vi "InstrumentControlExercises_MichaelVasmerDavidWise.vi"() -> ()   [LabVIEW 2012]
doc: "This example shows how to configure a measurement and take a reading."
uses:
  Program Files/National Instruments/LabVIEW 2014/instr.lib/Keithley 24XX/Keithley 24XX.lvlib
  <vilib>/express/express arith-compare/Formula/XNode/ExpressFormulaBlockNode.xnode
  Control2_MichaelVasmerDavidWise.ctl
  He3_Tlogger_Global 1.vi
  Control3_MichaelVasmerDavidWise.ctl
  Program Files/National Instruments/LabVIEW 2014/instr.lib/Stanford Research 830/Stanford Research 830.lvlib
  Program Files/National Instruments/LabVIEW 2014/instr.lib/Keithley 24XX/Public/Data/Read (Single Point).vi
  Program Files/National Instruments/LabVIEW 2014/instr.lib/Stanford Research 830/Public/Data/Read (All Parameters).vi
  <vilib>/Utility/file.llb/Write To Spreadsheet File (string).vi
  <vilib>/Utility/file.llb/Write To Spreadsheet File (DBL).vi
panel:
  out "T 2":dbl
  out "T 1":dbl
  out "Resistance(T) vs Time":dbl(graph)
  out "Resistance(B) vs Time":dbl(graph)
  out "V_output_Y_channel":dbl
  out "V_output_X_channel":dbl
  in  "R Series Value":dbl=100000.0
  in  "File String Template 2":string
  in  "File String Template":string
  in  "True  = R(B)\nFalse = R(T)":bool
  in  "Lock In On (default false)":bool
  out "Outer State Machine":T1=enum."Idle"
  in  "Force Measurement":bool
  out "Inner State Machine":T2=enum."Open File"
  out "I_AC Amplitude (A)":dbl=1.0
  in  "Keithley on (default false)":bool
  out "Magnetic Field (T)":dbl
  in  "Internal Reference Frequency (1000 Hz)":dbl=1000.0
  in  "Sine Output Amplitude (1 V)":dbl=1.0
  in  "Sensitivity (26: 1 V/uA)":i8(ring)=26 items=["Auto Gain"=-1, "2 nV/fA"=0, "5 nV/fA"=1, "10 nV/fA"=2, "20 nV/fA"=3, "50 nV/fA"=4, "100 nV/fA"=5, "200 nV/fA"=6, "500 nV/fA"=7, "1 uV/pA"=8, "2 uV/pA"=9, "5 uV/pA"=10, "10 uV/pA"=11, "20 uV/pA"=12, "50 uV/pA"=13, "100 uV/pA"=14, "200 uV/pA"=15, "500 uV/pA"=16, "1 mV/nA"=17, "2 mV/nA"=18, "5 mV/nA"=19, "10 mV/nA"=20, "20 mV/nA"=21, "50 mV/nA"=22, "100 mV/nA"=23, "200 mV/nA"=24, "500 mV/mA"=25, "1 V/uA"=26]
  in  "Dynamic Reserve (2: Low Noise)":i8(ring)=2 items=["High Reserve"=0, "Normal"=1, "Low Noise"=2, "Auto Reserve"=-1]
  in  "Reference Source (1: Internal)":u16(ring)=1 items=["External", "Internal"]
  in  "Input Coupling (0: AC)":u16(ring) items=["AC", "DC"]
  in  "Input Connection (0: Single-Ended Voltage)":u16(ring) items=["Single-Ended Voltage", "Differential Voltage", "1 MOhm Current Gain", "100 MOhm Current Gain"]
  in  "VISA resource name Lock-In":refnum<visa-resource-name>
  in  "Stop Sweep R(T)":bool
  in  "Sweep R(T)":bool
  out "Temperature (K)":dbl
  in  "Shutdown":bool
  in  "B Max\n|B|<0.0716":dbl
  in  "Sweep R(B)":bool
  in  "Steps":dbl
  out "Field too high error":string
  in  "Compliance  Level (0.1)":dbl=0.1
  out "Resistance":sgl
  out "Current":sgl
  out "Voltage":sgl
  in  "Enable Resistance Auto Range (T:Enable)":bool=TRUE
  in  "Enable Current Auto Range (T:Enable)":bool=TRUE
  in  "Enable Voltage Auto Range (T:Enable)":bool=TRUE
  in  "Resistance Manual Range (1.0)":dbl=1.0
  in  "Current Manual Range (1.0)":dbl=1.0
  in  "Voltage Manual Range (1.0)":dbl=1.0
  in  "Serial Configuration":T3={"Baud Rate"=9600, "Parity"=0, "Data Bits"=8, "Stop Bits"=10, "Flow Control"=0} {"Flow Control" items=["None", "XON/XOFF", "RTS/CTS", "XON/XOFF & RTS/CTS", "DTR/DSR", "XON/XOFF & DTR/DSR"]; "Stop Bits" items=["1.0"=10, "1.5"=15, "2.0"=20]; "Data Bits" items=["7"=7, "8"=8]; "Parity" items=["None", "Odd", "Even", "Mark", "Space"]; "Baud Rate" items=["300"=300, "600"=600, "1200"=1200, "2400"=2400, "4800"=4800, "9600"=9600, "19200"=19200]}
  in  "VISA resource name Kiethley":refnum<visa-resource-name>
  # "Keithley Settings"
  # "Voltage Range Settings"
  # "Current Range Settings"
  # "Resistance Range Settings"
  # "Keithley Output"
  # "SR830 Lock In Settings"
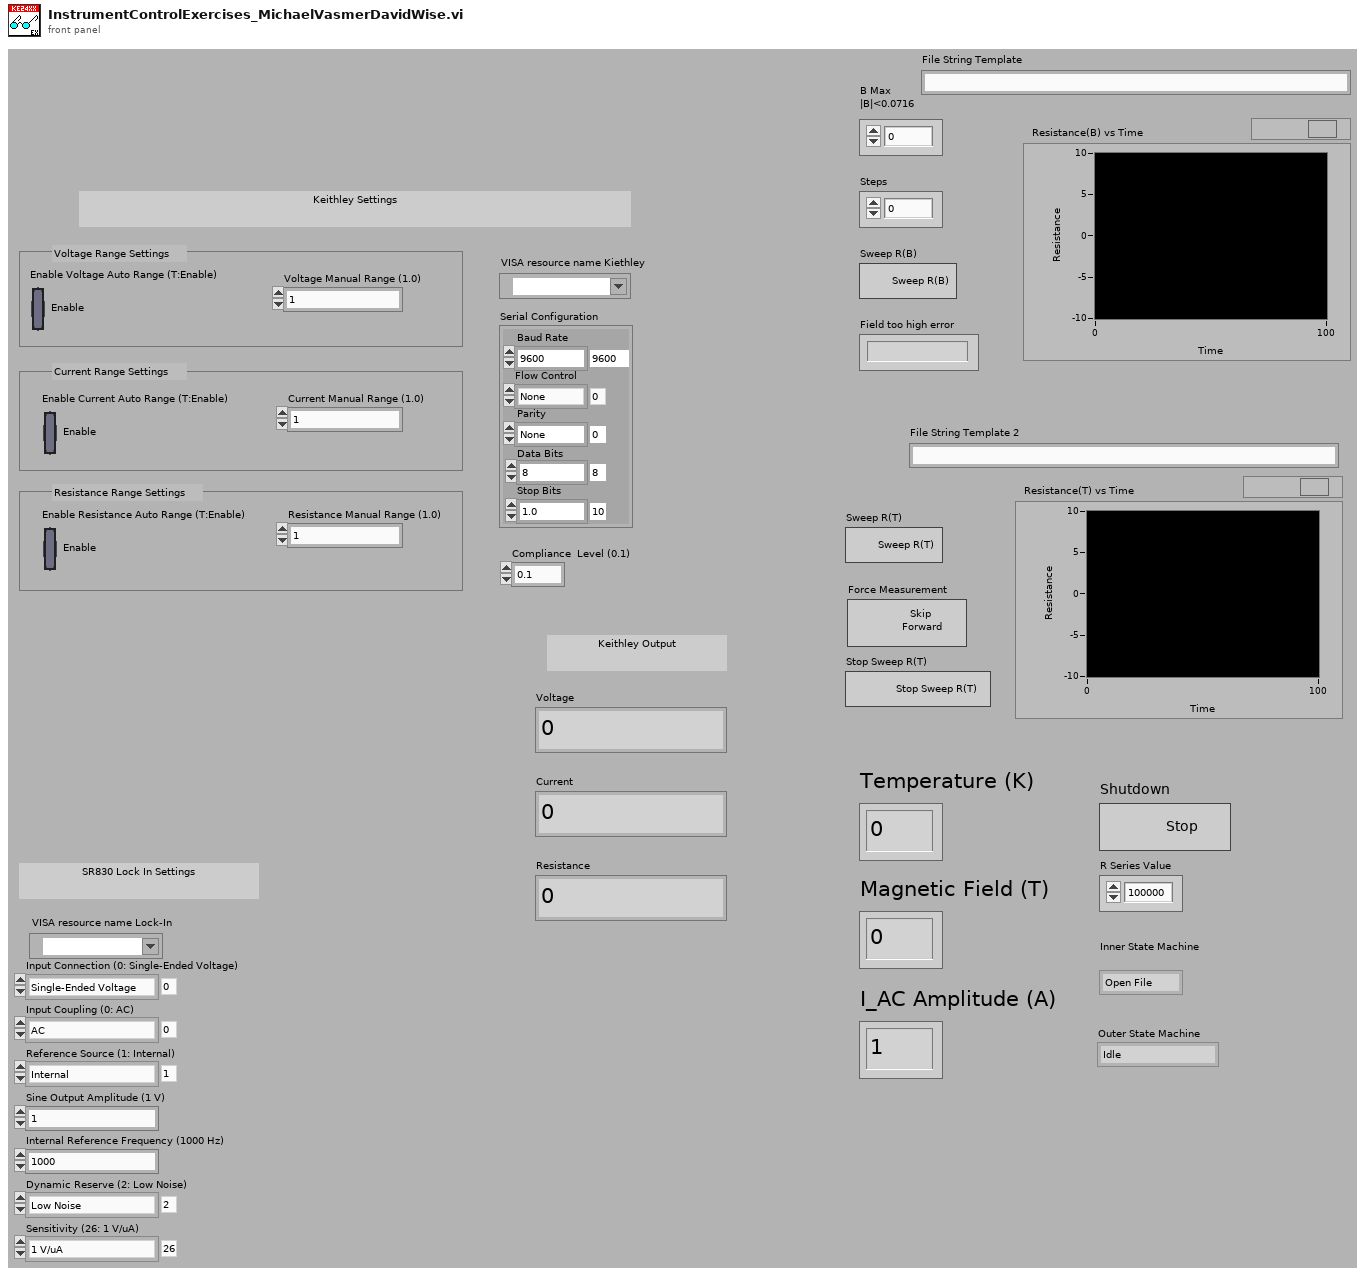
[diagram p1: front panel]
types:
  T1 = typedef "Control2_MichaelVasmerDavidWise.ctl" = enum16{"Write File", "Open File", "Shutdown All", "Shutdown Lock in", "Read R(T)", "Init Lock In", "Increment", "Shutdown Keithley", "Idle", "Exit", "Read R(B)", "Set B", "Init Keithley"}
  T2 = typedef "Control3_MichaelVasmerDavidWise.ctl" = enum16{"Write File", "Open File", "Read T 2", "Idle", "Read Lockin", "Read T"}
  T3 = cluster{"Baud Rate":u32, "Parity":u16, "Data Bits":u16, "Stop Bits":u16, "Flow Control":u16}
  T4 = cluster{"X-Value":dbl, "Y-Value":dbl, "R-Value":dbl, "Theta-Value":dbl, "Aux In 1 Value":dbl, "Aux In 2 Value":dbl, "Aux In 3 Value":dbl, "Aux In 4 Value":dbl, "Reference Frequency":dbl, "Channel 1 Display":dbl, "Channel 2 Display":dbl}
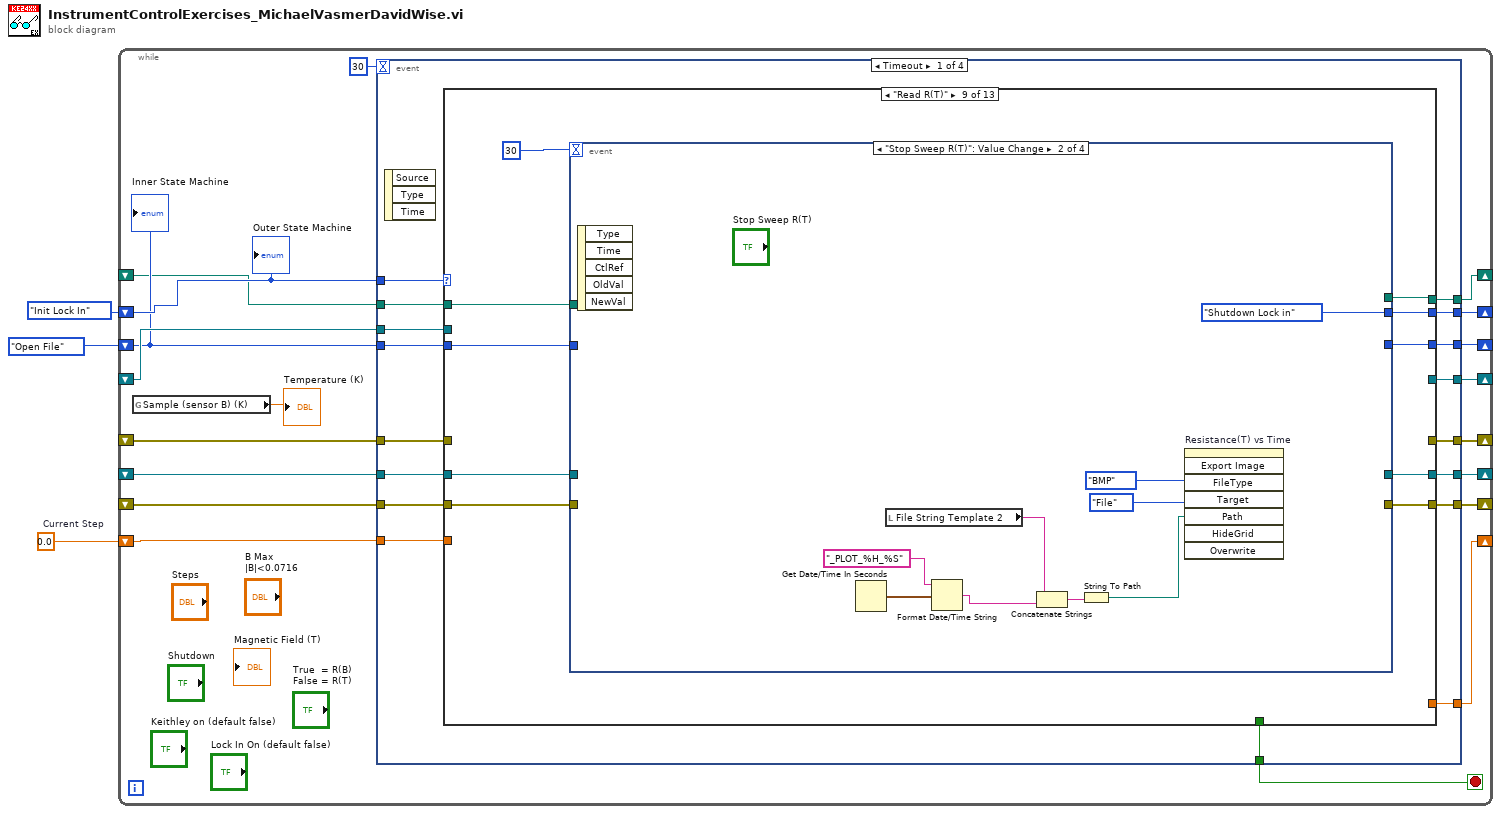
[diagram p0: block diagram]
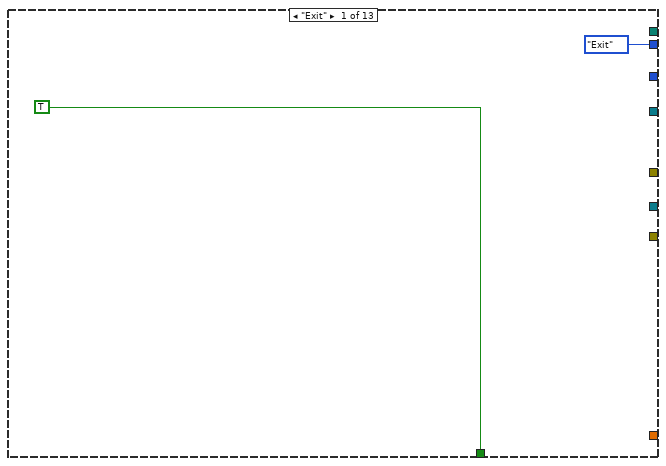
[diagram p2: hidden frame]
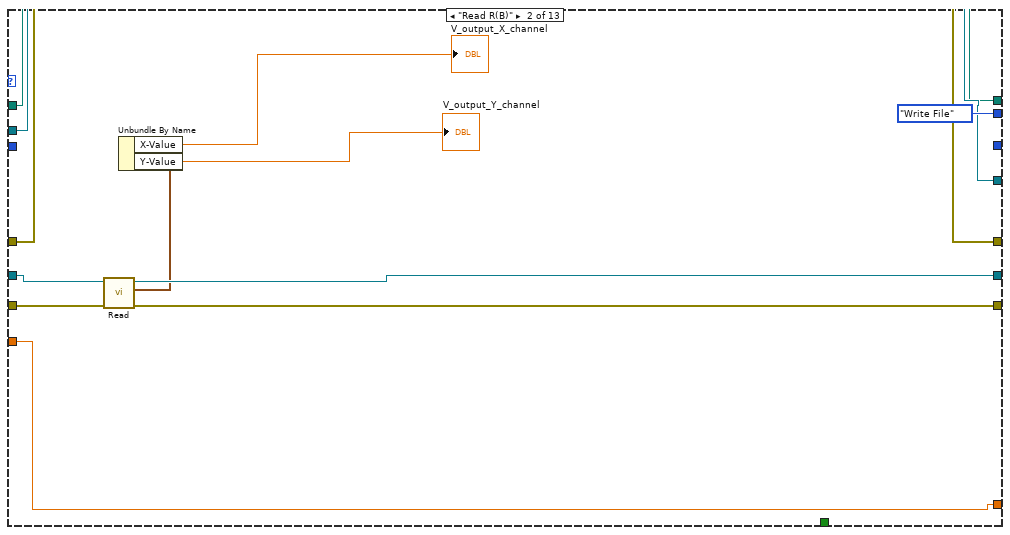
[diagram p3: hidden frame]
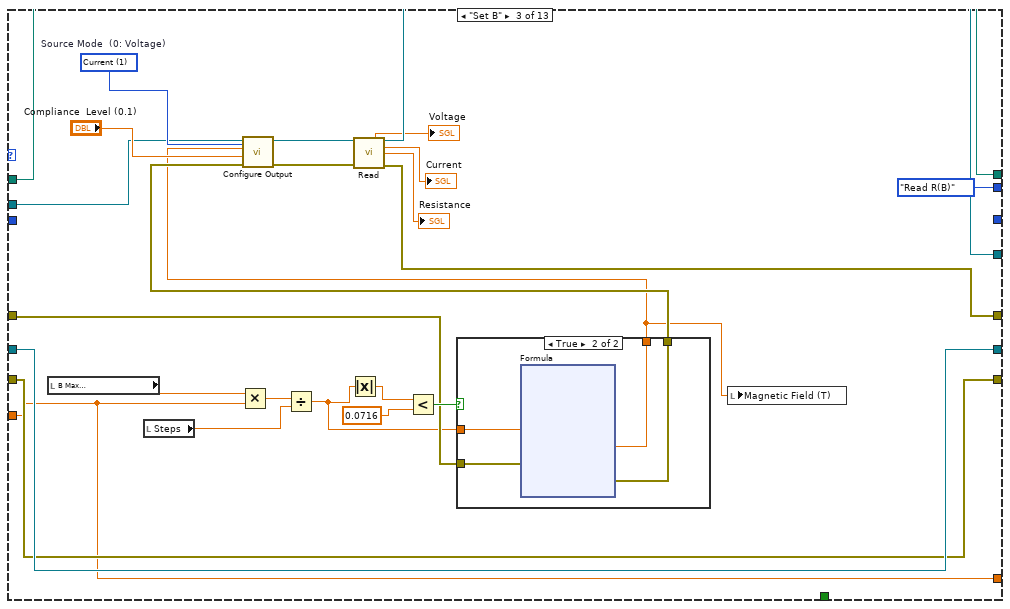
[diagram p4: hidden frame]
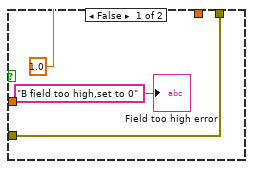
[diagram p5: hidden frame]
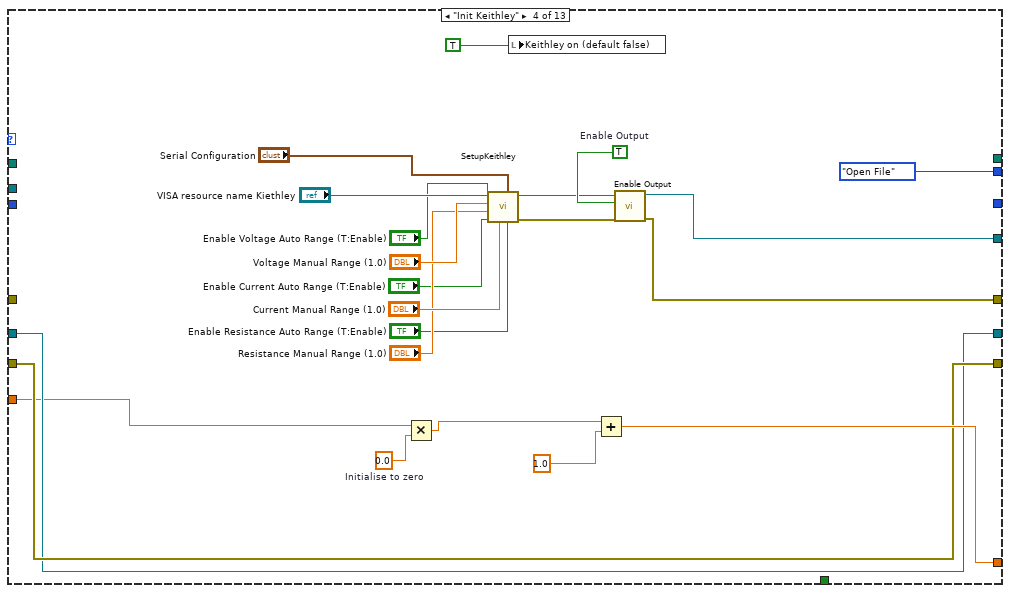
[diagram p6: hidden frame]
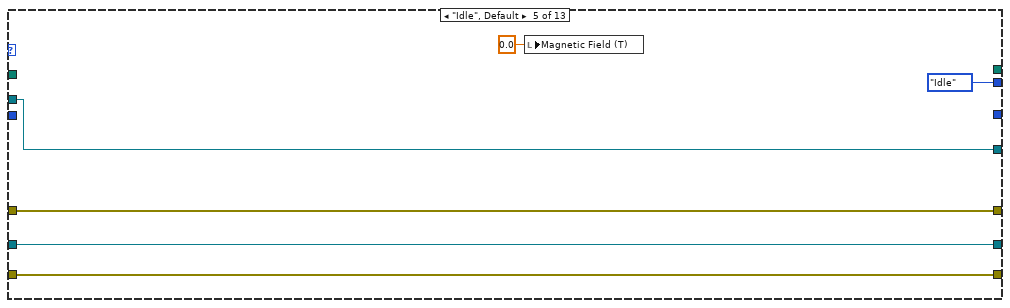
[diagram p7: hidden frame]
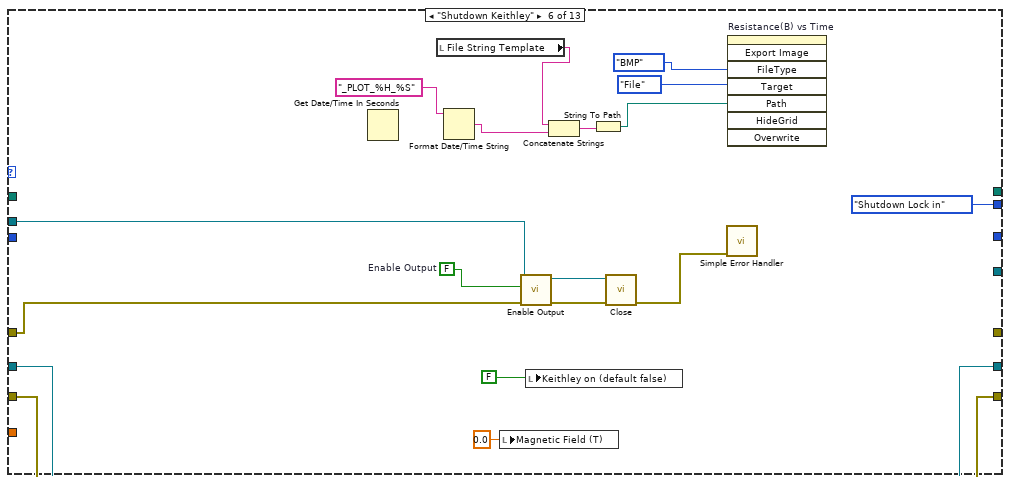
[diagram p8: hidden frame]
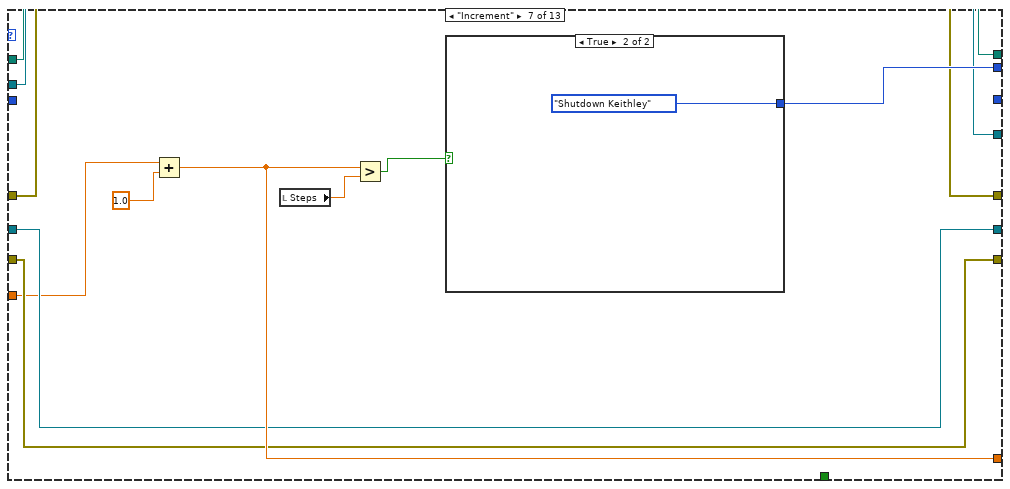
[diagram p9: hidden frame]
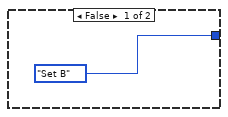
[diagram p10: hidden frame]
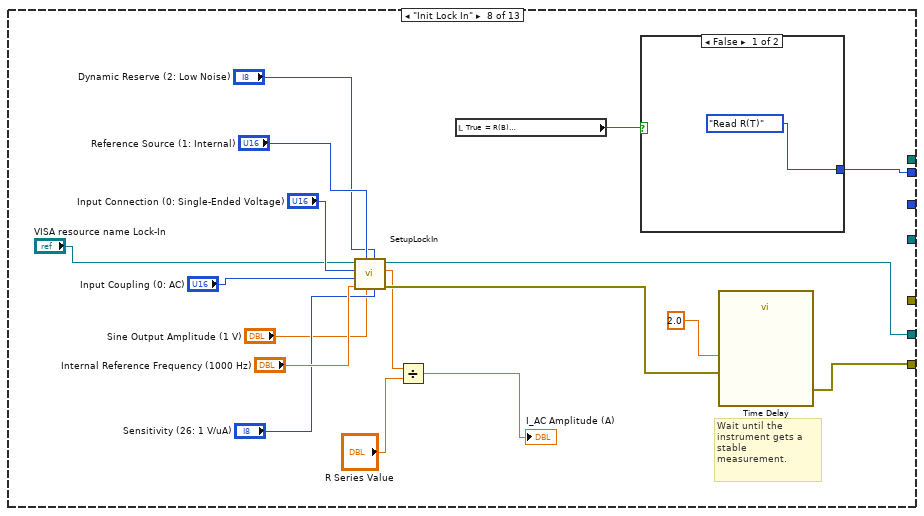
[diagram p11: hidden frame]
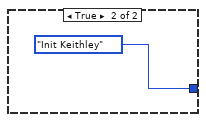
[diagram p12: hidden frame]
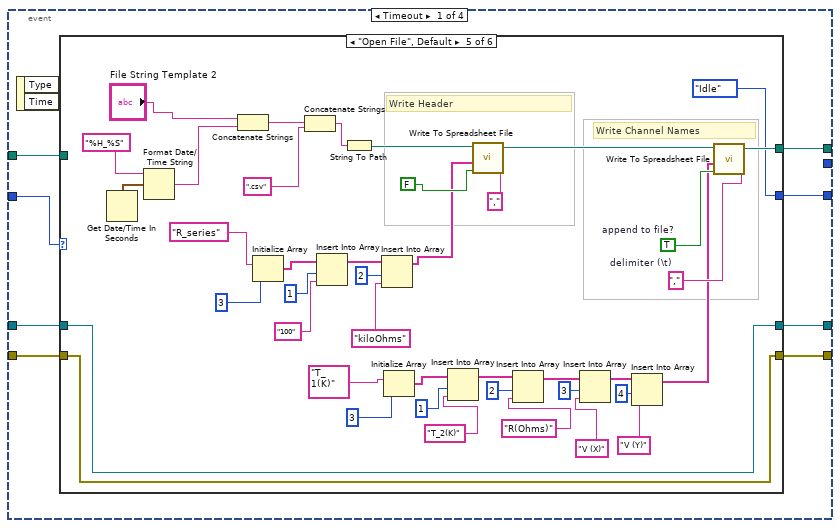
[diagram p13: hidden frame]
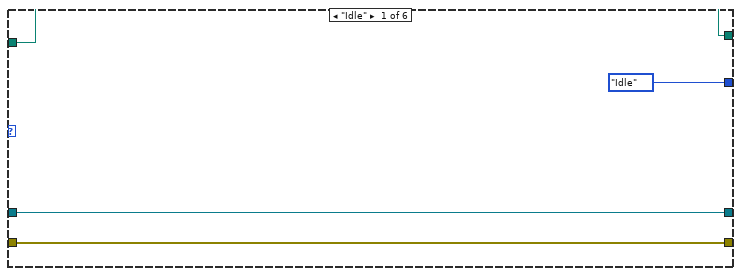
[diagram p14: hidden frame]
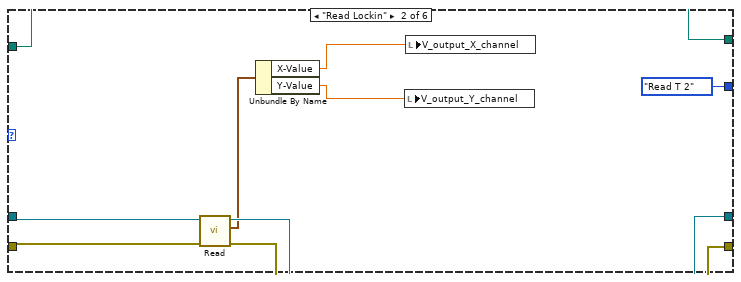
[diagram p15: hidden frame]
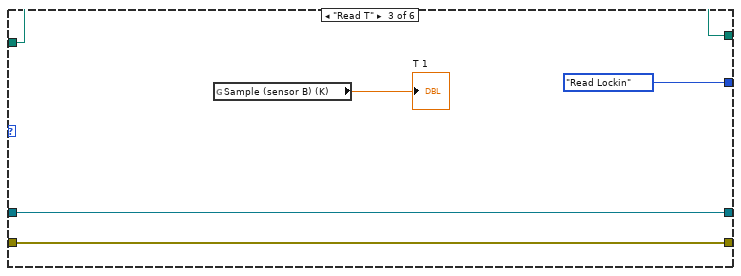
[diagram p16: hidden frame]
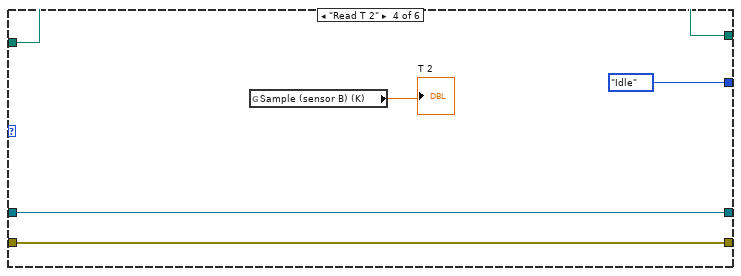
[diagram p17: hidden frame]
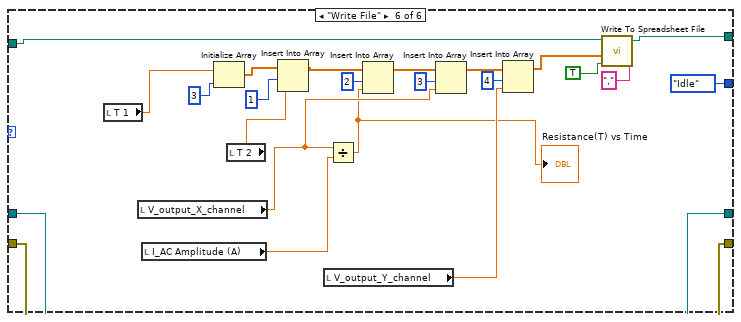
[diagram p18: hidden frame]
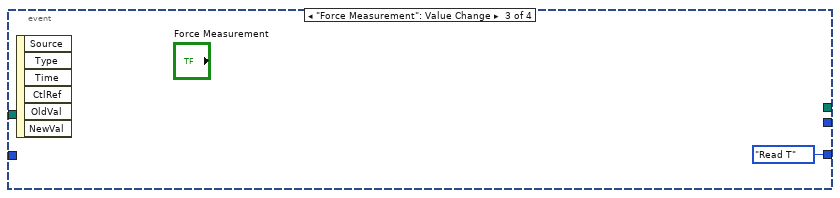
[diagram p19: hidden frame]
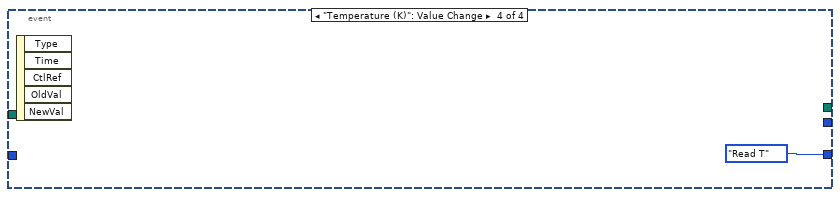
[diagram p20: hidden frame]
diagram:
  w2 = 0.0  # Current Step
  n1 = while {
    shift-right: [w21] -> _
    shift-left: Control2_MichaelVasmerDavidWise."Init Lock In" -> [w22]
    shift-right: [w20] -> _
    shift-left: _ -> [w17]
    shift-right: [w19] -> _
    shift-left: _ -> [w16]
    shift-right: [w14] -> _
    shift-left: w2 -> [w4]
    shift-right: [w13] -> _
    shift-left: Control3_MichaelVasmerDavidWise."Open File" -> [w7]
    shift-right: [w12] -> _
    shift-left: _ -> [w9]
    shift-right: [w11] -> _
    shift-left: _ -> [w10]
    shift-right: [w6] -> _
    shift-left: _ -> [w5]
    stop <- w15 stop-if-true
    n2 = global read "He3_Tlogger_Global 1.vi" "Sample (sensor B) (K)"() -> (→"Temperature (K)":dbl)
    n3 = event shown="[0] Timeout" {
      selector: _ -> [_ _ _ _]
      dyn-events: _ -> [_ _ _ _]
      timeout: 30 -> [_ _ _ _]
      tunnel: w22 -> [w39 _ _ _]
      tunnel: [w38 Control2_MichaelVasmerDavidWise."Shutdown All" Control2_MichaelVasmerDavidWise."Init Lock In" Control2_MichaelVasmerDavidWise."Init Lock In"] -> w21
      tunnel: [w37 _ _ _] -> w20
      tunnel: [w36 _ _ _] -> w19
      tunnel: w17 -> [w35 _ _ _]
      tunnel: w16 -> [w34 _ _ _]
      tunnel: [w33 _ _ _] -> w15
      tunnel: [w32 _ _ _] -> w14
      tunnel: w7 -> [w31 _ _ _]
      tunnel: [w30 _ _ _] -> w13
      tunnel: [w29 _ _ _] -> w12
      tunnel: [w28 _ _ _] -> w11
      tunnel: w10 -> [w27 _ _ _]
      tunnel: w9 -> [w26 _ _ _]
      tunnel: [w25 _ _ _] -> w6
      tunnel: w5 -> [w24 _ _ _]
      tunnel: w4 -> [w23 _ _ _]
      event Timeout {
        n4 = event-data() -> ()  [unwired: 1 in, 3 out]
        n5 = case shown="\"Read R(T)\"" w39 {
          tunnel: [Control2_MichaelVasmerDavidWise."Exit" Control2_MichaelVasmerDavidWise."Write File" Control2_MichaelVasmerDavidWise."Read R(B)" Control2_MichaelVasmerDavidWise."Open File" Control2_MichaelVasmerDavidWise."Idle" Control2_MichaelVasmerDavidWise."Shutdown Lock in" w148 w162 w178 Control2_MichaelVasmerDavidWise."Exit" _ Control2_MichaelVasmerDavidWise."Set B" Control2_MichaelVasmerDavidWise."Increment"] -> w38
          tunnel: [_ w48 w59 w107 w120 _ w146 _ _ _ _ _ w370] -> w37
          tunnel: [_ w47 w60 w99 w121 _ w145 _ _ _ _ _ w371] -> w36
          tunnel: w35 -> [_ w48 w63 _ w120 w134 w146 _ _ w291 _ _ w370]
          tunnel: w34 -> [_ w47 w61 _ w121 w138 w145 _ _ w292 _ _ w371]
          tunnel: [TRUE _ _ _ _ _ _ _ _ _ _ _ _] -> w33
          tunnel: [_ w42 w54 w103 _ _ w147 _ _ _ _ w310 w351] -> w32
          tunnel: w31 -> [_ _ _ _ _ _ _ _ w180 _ _ _ _]
          tunnel: [_ _ _ _ _ _ _ _ w179 _ _ _ _] -> w30
          tunnel: [_ w52 w67 w96 w117 w129 w143 w161 w174 _ _ _ w372] -> w29
          tunnel: [_ w51 w66 w97 w116 w130 w144 w159 w175 _ _ _ w373] -> w28
          tunnel: w27 -> [_ w50 w66 w97 w116 w130 w144 _ w177 w289 w307 _ w373]
          tunnel: w26 -> [_ w46 w67 w96 w117 w129 w143 _ w176 w290 w308 _ w372]
          tunnel: [_ w45 w55 _ _ _ w141 _ w173 _ _ w322 _] -> w25
          tunnel: w24 -> [_ w45 w55 _ _ _ w141 _ w172 _ _ _ w367]
          tunnel: w23 -> [_ w42 w54 w94 _ _ w140 _ _ _ _ w310 w351]
          frame "Exit" {
          }
          frame "Read R(B)" {
            n6 = call-poly "Read.vi"("error in (no error)"=w50, "VISA resource name"=w46) -> ("error out"=w51:errorcluster, "Parameter Values"=w49:T4, "VISA resource name out"=w52:refnum<visa-resource-name>)  [unwired: 7 in]
            n7 = Unbundle By Name(w49) -> ("X-Value"=→"V_output_X_channel":dbl, "Y-Value"=→"V_output_Y_channel":dbl)
          }
          frame "Set B" {
            w73 = u16 1 items=["Voltage", "Current"]  # Source Mode  (0: Voltage)
            n8 = local read "B Max\n|B|<0.0716"() -> (w70:dbl)
            n9 = local read "Steps"() -> (w68:dbl)
            n10 = Multiply(x=w70, y=w54) -> (x*y=w69:dbl)
            n11 = Divide(x=w69, y=w68) -> (x/y=w56:dbl)
            n12 = Absolute Value(x=w56) -> (abs(x)=w57:dbl)
            n13 = Less?(x=w57, y=0.0716 ("x")) -> (x < y?=w72:bool)
            n14 = case shown="True" w72 {
              tunnel: w56 -> [_ w85]
              tunnel: [1.0 ("x") w84] -> w62
              tunnel: w61 -> [w80 w83]
              tunnel: [w80 w82] -> w65
              frame False {
                "Field too high error" <- "B field too high,set to 0" ("String")
              }
              frame True {
                n15 = xnode "Formula"("X1"=w85, "error in (no error)"=w83) -> ("Result"=w84:dbl, "error out"=w82:errorcluster)
              }
            }
            n16 = call "Configure Output.vi"("Source Mode  (0: Voltage)"=w73, "error in (no error)"=w65, "Compliance  Level (0.1)"="Compliance  Level (0.1)", "Output Level (0)"=w62, "VISA resource name"=w63) -> ("error out"=w74:errorcluster, "VISA resource name out"=w75:refnum<visa-resource-name>)  [unwired: 5 in]
            n17 = call-poly "Read.vi"("VISA resource name"=w75, "error in (no error)"=w74) -> ("Voltage"=→"Voltage":sgl, "VISA resource name out"=w59:refnum<visa-resource-name>, "Current"=→"Current":sgl, "Resistance"=→"Resistance":sgl, "error out"=w60:errorcluster)  [unwired: 7 in, 2 out]
            n18 = local write "Magnetic Field (T)"(w62) -> ()
          }
          frame "Init Keithley" {
            w105 = 0.0  # Initialise to zero
            w108 = TRUE  # Enable Output
            n19 = Multiply(x=w94, y=w105) -> (x*y=w106:dbl)
            n20 = call "SetupKeithley.vi"("Enable Resistance Auto Range (T:Enable)"="Enable Resistance Auto Range (T:Enable)", "Serial Configuration"="Serial Configuration", "Current Manual Range (1.0)"="Current Manual Range (1.0)", "Enable Voltage Auto Range (T:Enable)"="Enable Voltage Auto Range (T:Enable)", "Enable Current Auto Range (T:Enable)"="Enable Current Auto Range (T:Enable)", "Resistance Manual Range (1.0)"="Resistance Manual Range (1.0)", "Voltage Manual Range (1.0)"="Voltage Manual Range (1.0)", "VISA Refnum in"="VISA resource name Kiethley") -> ("error out"=w100:errorcluster, "VISA Refnum out"=w98:refnum<visa-resource-name>)  [unwired: 2 in]
            n21 = local write "Keithley on (default false)"(TRUE ("Keithley on")) -> ()
            n22 = Add(x=w106, y=1.0 ("x+y")) -> (x+y=w103:dbl)
            n23 = call "Enable Output.vi"("error in (no error)"=w100, "Enable Output (T: Enable)"=w108, "VISA resource name"=w98) -> ("error out"=w99:errorcluster, "VISA resource name out"=w107:refnum<visa-resource-name>)  [unwired: 7 in]
          }
          frame "Idle", Default {
            n24 = local write "Magnetic Field (T)"(0.0 ("Magnetic Field (T)")) -> ()
          }
          frame "Shutdown Keithley" {
            w131 = FALSE  # Enable Output
            n25 = Get Date/Time In Seconds() -> ()  [unwired: 1 out]
            n26 = local read "File String Template"() -> (w123:string)
            n27 = Format Date/Time String(time format string (%c)="_PLOT_%H_%S") -> (date/time string=w122:string)  [unwired: 2 in]
            n28 = local write "Magnetic Field (T)"(0.0 ("Magnetic Field (T)")) -> ()
            n29 = call "Enable Output.vi"("error in (no error)"=w138, "Enable Output (T: Enable)"=w131, "VISA resource name"=w134) -> ("error out"=w139:errorcluster, "VISA resource name out"=w133:refnum<visa-resource-name>)  [unwired: 7 in]
            n30 = local write "Keithley on (default false)"(FALSE ("Keithley on")) -> ()
            n31 = Concatenate Strings(w123, w122) -> (w126:string)
            n32 = String To Path(string=w126) -> (path=w125:path)
            n33 = call "Close.vi"("error in (no error)"=w139, "VISA resource name"=w133) -> ("error out"=w132:errorcluster)  [unwired: 9 in]
            n34 = call <vilib>:"Simple Error Handler.vi"("error in (no error)"=w132) -> ()  [unwired: 4 in, 5 out]
            n35 = invoke on="Resistance(B) vs Time" class="WFChart (strict)" method="Export Image"("FileType"=enum32{"BMP", "EPS", "EMF", "PICT"}."BMP" ("File Type"), "Target"=enum32{"File", "Clipboard"}."File", "Path"=w125) -> ()  [unwired: 5 in, 8 out]
          }
          frame "Increment" {
            n36 = Add(x=w140, y=1.0 ("x")) -> (x+y=w147:dbl)
            n37 = local read "Steps"() -> (w149:dbl)
            n38 = Greater?(x=w147, y=w149) -> (0:w142:bool)
            n39 = case shown="True" w142 {
              tunnel: [Control2_MichaelVasmerDavidWise."Set B" Control2_MichaelVasmerDavidWise."Shutdown Keithley"] -> w148
              frame False {
              }
              frame True {
              }
            }
          }
          frame "Init Lock In" {
            # "Wait until the instrument gets a stable measurement."
            n40 = call "SetupLockIn.vi"("Sensitivity (26: 1 V/uA)"="Sensitivity (26: 1 V/uA)", "Dynamic Reserve (2: Low Noise)"="Dynamic Reserve (2: Low Noise)", "Sine Output Amplitude (1 V)"="Sine Output Amplitude (1 V)", "Reference Source (1: Internal)"="Reference Source (1: Internal)", "Internal Reference Frequency (1000 Hz)"="Internal Reference Frequency (1000 Hz)", "Input Coupling (0: AC)"="Input Coupling (0: AC)", "Input Connection (0: Single-Ended Voltage)"="Input Connection (0: Single-Ended Voltage)", "VISA Refnum in"="VISA resource name Lock-In") -> ("error out"=w160:errorcluster, "V_AC Amplitude (A)"=w155:dbl, "VISA Refnum out"=w161:refnum<visa-resource-name>)  [unwired: 1 in]
            n41 = Divide(x=w155, y="R Series Value") -> (x/y=→"I_AC Amplitude (A)":dbl)
            n42 = local read "True  = R(B)\nFalse = R(T)"() -> (w156:bool)
            n43 = case shown="False" w156 {
              tunnel: [Control2_MichaelVasmerDavidWise."Read R(T)" Control2_MichaelVasmerDavidWise."Init Keithley"] -> w162
              frame False {
              }
              frame True {
              }
            }
            n44 = call "Time Delay"("error in (no error)"=w160, "Delay Time (s)"=2.0) -> ("error out"=w159:errorcluster)  [unwired: 9 in]
          }
          frame "Read R(T)" {
            n45 = event shown="[1] \"Stop Sweep R(T)\": Value Change" {
              selector: _ -> [_ _ _ _]
              dyn-events: _ -> [_ _ _ _]
              timeout: 30 -> [_ _ _ _]
              tunnel: w180 -> [w189 _ _ _]
              tunnel: [w188 _ Control3_MichaelVasmerDavidWise."Read T" Control3_MichaelVasmerDavidWise."Read T"] -> w179
              tunnel: [_ Control2_MichaelVasmerDavidWise."Shutdown Lock in" _ _] -> w178
              tunnel: w177 -> [w187 _ _ _]
              tunnel: w176 -> [w186 _ _ _]
              tunnel: [w185 _ _ _] -> w175
              tunnel: [w184 _ _ _] -> w174
              tunnel: [w183 _ _ _] -> w173
              tunnel: w172 -> [w182 _ _ _]
              event Timeout {
                n46 = event-data() -> ()  [unwired: 1 in, 2 out]
                n47 = case shown="\"Open File\", Default" w189 {
                  tunnel: [Control3_MichaelVasmerDavidWise."Idle" Control3_MichaelVasmerDavidWise."Read T 2" Control3_MichaelVasmerDavidWise."Read Lockin" Control3_MichaelVasmerDavidWise."Idle" Control3_MichaelVasmerDavidWise."Idle" Control3_MichaelVasmerDavidWise."Idle"] -> w188
                  tunnel: w187 -> [w191 w200 w205 w210 w217 w276]
                  tunnel: w186 -> [w192 w201 w206 w211 w216 w275]
                  tunnel: [w191 w199 w205 w210 w217 w276] -> w185
                  tunnel: [w192 w198 w206 w211 w216 w275] -> w184
                  tunnel: [w190 w194 w203 w208 w220 w272] -> w183
                  tunnel: w182 -> [w190 w194 w203 w208 _ w271]
                  frame "Idle" {
                  }
                  frame "Read Lockin" {
                    n48 = call-poly "Read.vi"("error in (no error)"=w200, "VISA resource name"=w201) -> ("error out"=w199:errorcluster, "Parameter Values"=w197:T4, "VISA resource name out"=w198:refnum<visa-resource-name>)  [unwired: 7 in]
                    n49 = Unbundle By Name(w197) -> ("X-Value"=w196:dbl, "Y-Value"=w195:dbl)
                    n50 = local write "V_output_Y_channel"(w195) -> ()
                    n51 = local write "V_output_X_channel"(w196) -> ()
                  }
                  frame "Read T" {
                    n52 = global read "He3_Tlogger_Global 1.vi" "Sample (sensor B) (K)"() -> (→"T 1":dbl)
                  }
                  frame "Read T 2" {
                    n53 = global read "He3_Tlogger_Global 1.vi" "Sample (sensor B) (K)"() -> (→"T 2":dbl)
                  }
                  frame "Open File", Default {
                    w252 = TRUE  # append to file?
                    w250 = ","  # delimiter (\t)
                    # "Write Header"
                    # "Write Channel Names"
                    n54 = Get Date/Time In Seconds() -> (seconds since 1Jan1904=w215:timestamp)
                    n55 = Format Date/Time String(time format string (%c)="%H_%S", seconds (now)=w215) -> (date/time string=w214:string)  [unwired: 1 in]
                    n56 = Concatenate Strings("File String Template 2", w214) -> (w247:string)
                    n57 = Initialize Array("R_series", 3 ("dimension size")) -> (w244:string[])
                    n58 = Concatenate Strings(w247, ".csv" ("string")) -> (w248:string)
                    n59 = Insert Into Array(array=w244, index=1, new element="100") -> (w243:string[])
                    n60 = String To Path(string=w248) -> (path=w249:path)
                    n61 = Insert Into Array(array=w243, index=2, new element="kiloOhms") -> (w236:string[])
                    n62 = Initialize Array("T_1(K)", 3 ("dimension size")) -> (w235:string[])
                    n63 = Insert Into Array(array=w235, index=1, new element="T_2(K)") -> (w234:string[])
                    n64 = call-poly <vilib>:"Write To Spreadsheet File.vi"("delimiter (\\t)"="," ("delimiter (\\t)"), "append to file? (new file:F)"=FALSE, "1D data"=w236, "file path (dialog if empty)"=w249) -> ("new file path (Not A Path if cancelled)"=w251:path)  [unwired: 3 in, 1 out]
                    n65 = Insert Into Array(array=w234, index=2, new element="R(Ohms)") -> (w223:string[])
                    n66 = Insert Into Array(array=w223, index=3, new element="V (X)") -> (w222:string[])
                    n67 = Insert Into Array(array=w222, index=4, new element="V (Y)") -> (w221:string[])
                    n68 = call-poly <vilib>:"Write To Spreadsheet File.vi"("delimiter (\\t)"=w250, "append to file? (new file:F)"=w252, "1D data"=w221, "file path (dialog if empty)"=w251) -> ("new file path (Not A Path if cancelled)"=w220:path)  [unwired: 3 in, 1 out]
                  }
                  frame "Write File" {
                    n69 = local read "T 1"() -> (w267:dbl)
                    n70 = local read "V_output_X_channel"() -> (w259:dbl)
                    n71 = local read "I_AC Amplitude (A)"() -> (w260:dbl)
                    n72 = Initialize Array(w267, 3 ("dimension size")) -> (w266:dbl[])
                    n73 = local read "T 2"() -> (w268:dbl)
                    n74 = Insert Into Array(array=w266, index=1, new element=w268) -> (w264:dbl[])
                    n75 = local read "V_output_Y_channel"() -> (w261:dbl)
                    n76 = Divide(x=w259, y=w260) -> (x/y=w254:dbl)
                    "Resistance(T) vs Time" <- w254
                    n77 = Insert Into Array(array=w264, index=2, new element=w254) -> (w263:dbl[])
                    n78 = Insert Into Array(array=w263, index=3, new element=w259) -> (w262:dbl[])
                    n79 = Insert Into Array(array=w262, index=4, new element=w261) -> (w255:dbl[])
                    n80 = call-poly <vilib>:"Write To Spreadsheet File.vi"("delimiter (\\t)"="," ("delimiter (\\t)"), "append to file? (new file:F)"=TRUE, "1D data"=w255, "file path (dialog if empty)"=w271) -> ("new file path (Not A Path if cancelled)"=w272:path)  [unwired: 3 in, 1 out]
                  }
                }
              }
              event "Stop Sweep R(T)": Value Change {
                n81 = event-data() -> ()  [unwired: 1 in, 5 out]
                n82 = Get Date/Time In Seconds() -> (seconds since 1Jan1904=w277:timestamp)
                n83 = local read "File String Template 2"() -> (w279:string)
                n84 = Format Date/Time String(time format string (%c)="_PLOT_%H_%S", seconds (now)=w277) -> (date/time string=w280:string)  [unwired: 1 in]
                n85 = Concatenate Strings(w279, w280) -> (w282:string)
                n86 = String To Path(string=w282) -> (path=w278:path)
                n87 = invoke on="Resistance(T) vs Time" class="WFChart (strict)" method="Export Image"("FileType"=enum32{"BMP", "EPS", "EMF", "PICT"}."BMP" ("File Type"), "Target"=enum32{"File", "Clipboard"}."File", "Path"=w278) -> ()  [unwired: 5 in, 8 out]
              }
              event "Force Measurement": Value Change {
                n88 = event-data() -> ()  [unwired: 1 in, 6 out]
              }
              event "Temperature (K)": Value Change {
                n89 = event-data() -> ()  [unwired: 1 in, 5 out]
              }
            }
          }
          frame "Shutdown All" {
            n90 = local read "Keithley on (default false)"() -> (w293:bool)
            n91 = local read "Lock In On (default false)"() -> (w288:bool)
            n92 = case shown="True" w293 {
              tunnel: w292 -> [_ w300]
              tunnel: w291 -> [_ w299]
              frame False {
              }
              frame True {
                w305 = FALSE  # Enable Output
                n93 = call "Enable Output.vi"("error in (no error)"=w300, "Enable Output (T: Enable)"=w305, "VISA resource name"=w299) -> ("error out"=w304:errorcluster, "VISA resource name out"=w302:refnum<visa-resource-name>)  [unwired: 7 in]
                n94 = local write "Keithley on (default false)"(FALSE ("Keithley on")) -> ()
                n95 = call "Close.vi"("error in (no error)"=w304, "VISA resource name"=w302) -> ("error out"=w303:errorcluster)  [unwired: 9 in]
                n96 = call <vilib>:"Simple Error Handler.vi"("error in (no error)"=w303) -> ()  [unwired: 4 in, 5 out]
              }
            }
            n97 = case shown="True" w288 {
              tunnel: w290 -> [_ w297]
              tunnel: w289 -> [_ w296]
              frame False {
              }
              frame True {
                n98 = call "Close.vi"("error in (no error)"=w296, "VISA resource name"=w297) -> ("error out"=w298:errorcluster)  [unwired: 9 in]
                n99 = call <vilib>:"Simple Error Handler.vi"("error in (no error)"=w298) -> ()  [unwired: 4 in, 5 out]
                n100 = local write "Lock In On (default false)"(FALSE ("Lock In On (default false)")) -> ()
              }
            }
          }
          frame "Shutdown Lock in" {
            n101 = call "Close.vi"("error in (no error)"=w307, "VISA resource name"=w308) -> ("error out"=w309:errorcluster)  [unwired: 9 in]
            n102 = local write "Lock In On (default false)"(FALSE ("Lock In On (default false)")) -> ()
            n103 = call <vilib>:"Simple Error Handler.vi"("error in (no error)"=w309) -> ()  [unwired: 4 in, 5 out]
          }
          frame "Open File" {
            w348 = TRUE  # append to file?
            w346 = ","  # delimiter (\t)
            # "Write Header"
            # "Write Channel Names"
            n104 = Get Date/Time In Seconds() -> (seconds since 1Jan1904=w313:timestamp)
            n105 = Format Date/Time String(time format string (%c)="%H_%S", seconds (now)=w313) -> (date/time string=w312:string)  [unwired: 1 in]
            n106 = Concatenate Strings("File String Template", w312) -> (w342:string)
            n107 = Initialize Array("R_series", 3 ("dimension size")) -> (w339:string[])
            n108 = Concatenate Strings(w342, ".csv" ("string")) -> (w343:string)
            n109 = Insert Into Array(array=w339, index=1, new element="100") -> (w338:string[])
            n110 = String To Path(string=w343) -> (path=w345:path)
            n111 = Insert Into Array(array=w338, index=2, new element="kiloOhms") -> (w331:string[])
            n112 = Initialize Array("B(T)", 3 ("dimension size")) -> (w330:string[])
            n113 = Insert Into Array(array=w330, index=1, new element="R(Ohms)") -> (w329:string[])
            n114 = call-poly <vilib>:"Write To Spreadsheet File.vi"("delimiter (\\t)"="," ("delimiter (\\t)"), "append to file? (new file:F)"=FALSE, "1D data"=w331, "file path (dialog if empty)"=w345) -> ("new file path (Not A Path if cancelled)"=w347:path)  [unwired: 3 in, 1 out]
            n115 = Insert Into Array(array=w329, index=2, new element="T(K)") -> (w316:string[])
            n116 = Insert Into Array(array=w316, index=3, new element="V (X)") -> (w315:string[])
            n117 = Insert Into Array(array=w315, index=4, new element="V (Y)") -> (w314:string[])
            n118 = call-poly <vilib>:"Write To Spreadsheet File.vi"("delimiter (\\t)"=w346, "append to file? (new file:F)"=w348, "1D data"=w314, "file path (dialog if empty)"=w347) -> ("new file path (Not A Path if cancelled)"=w322:path)  [unwired: 3 in, 1 out]
          }
          frame "Write File" {
            n119 = local read "Magnetic Field (T)"() -> (w356:dbl)
            n120 = local read "V_output_Y_channel"() -> (w350:dbl)
            n121 = local read "V_output_X_channel"() -> (w353:dbl)
            n122 = local read "Temperature (K)"() -> (w355:dbl)
            n123 = local read "I_AC Amplitude (A)"() -> (w354:dbl)
            n124 = Initialize Array(w356, 3 ("dimension size")) -> (w366:dbl[])
            n125 = Divide(x=w353, y=w354) -> (x/y=w352:dbl)
            "Resistance(B) vs Time" <- w352
            n126 = Insert Into Array(array=w366, index=1, new element=w352) -> (w365:dbl[])
            n127 = Insert Into Array(array=w365, index=2, new element=w355) -> (w359:dbl[])
            n128 = Insert Into Array(array=w359, index=3, new element=w353) -> (w358:dbl[])
            n129 = Insert Into Array(array=w358, index=4, new element=w350) -> (w357:dbl[])
            n130 = call-poly <vilib>:"Write To Spreadsheet File.vi"("delimiter (\\t)"="," ("delimiter (\\t)"), "append to file? (new file:F)"=TRUE, "1D data"=w357, "file path (dialog if empty)"=w367) -> ()  [unwired: 3 in, 2 out]
          }
        }
      }
      event "Shutdown": Value Change {
        n131 = event-data() -> ()  [unwired: 1 in, 6 out]
      }
      event "Sweep R(T)": Value Change {
        n132 = event-data() -> ()  [unwired: 1 in, 6 out]
        n133 = local write "True  = R(B)\nFalse = R(T)"(FALSE ("True  = R(B)\nFalse = R(T)")) -> ()
      }
      event "Sweep R(B)": Value Change {
        n134 = event-data() -> ()  [unwired: 1 in, 6 out]
        n135 = local write "True  = R(B)\nFalse = R(T)"(TRUE ("True  = R(B)\nFalse = R(T)")) -> ()
      }
    }
    "Inner State Machine" <- w7
    "Outer State Machine" <- w22
  }
